vi "Lab3_4Var.vi"() -> ()   [LabVIEW 2022 SP3]
uses:
  71a54693-e4ba-4cbb-9a36-66ab201ab688.vi
  <vilib>/regexp/Match Regular Expression.xnode
panel:
  in  "String":string
  out "Array":i64[](array[numeric])
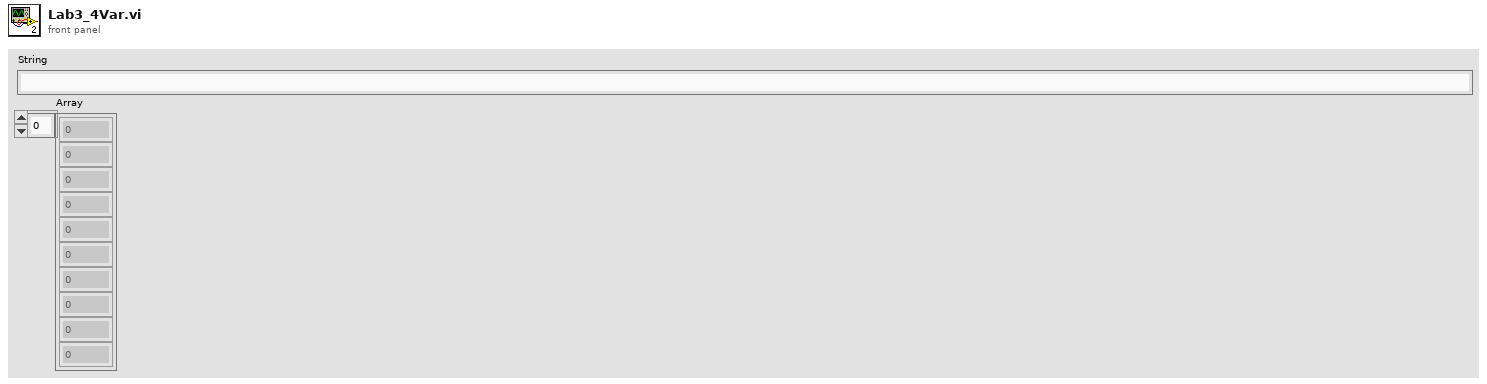
[diagram p1: front panel]
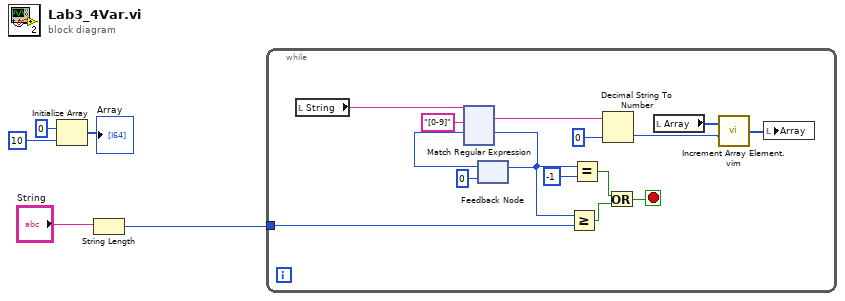
[diagram p0: block diagram]
diagram:
  n1 = Initialize Array(i64 0 ("element"), 10 ("dimension size")) -> (→"Array":i64[])
  n2 = String Length(string="String") -> (length=w1:i32)
  n3 = while {
    tunnel: w1 -> [w18]
    stop <- w16 stop-if-true
    n4 = local read "String"() -> (w14:string)
    n5 = feedback #1(0 ("offset past match")) -> (w20:i32)
    n6 = xnode "Match Regular Expression"("input string"=w14, "regular expression"="[0-9]", "offset (0)"=w20) -> ("whole match"=w12:string, "offset past match"=w7:i32)  [unwired: 3 in, 3 out]
    n7 = feedback-in #1(w7) -> ()
    n8 = Greater Or Equal?(x=w7, y=w18) -> (x >= y?=w17:bool)
    n9 = Equal?(x=w7, y=-1) -> (x = y?=w8:bool)
    n10 = Decimal String To Number(string=w12, default (0L)=i8 0 ("default (0 I32)")) -> (number=w10:i8)  [unwired: 1 in, 1 out]
    n11 = Or(x=w8, y=w17) -> (x .or. y?=w16:bool)
    n12 = local read "Array"() -> (w11:i64[])
    n13 = call "Increment Array Element.vim"("index"=w10, "array in"=w11) -> ("array out"=w9:i64[])
    n14 = local write "Array"(w9) -> ()
  }
